vi "AV Write Array.vi"(8 "error in":errorcluster, 10 "Actual Value":dbl[](array[numeric]), 11 "Current Actual Value in":refnum<class "Current Actual Value.lvclass">) -> (0 "error out":errorcluster, 3 "Current Actual Value out":refnum<class "Current Actual Value.lvclass">)   [LabVIEW 2023, in "Current Actual Value.lvclass"]
uses:
  Current Actual Value.lvclass
  Current Actual Value.lvclass/Current Actual Value.ctl
  Parents/Actual Value/Actual Value.lvclass
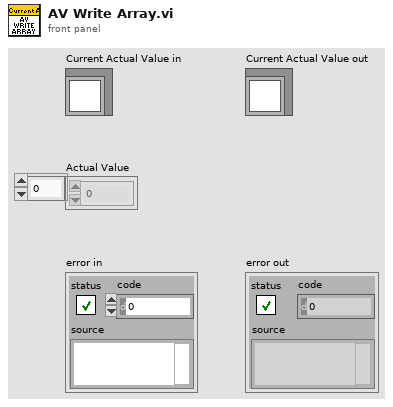
[diagram p1: front panel]
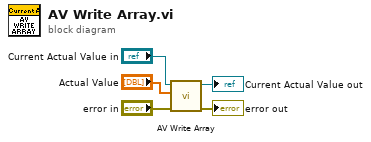
[diagram p0: block diagram]
diagram:
  n1 = call-parent "AV Write Array.vi"("error in"="error in", "Actual Value"="Actual Value", "Actual Value in"="Current Actual Value in") -> ("error out"=→"error out":errorcluster, "Actual Value out"=→"Current Actual Value out":refnum<class "Current Actual Value.lvclass">)  [unwired: 7 in]
